vi "Façade 1.vi"(0 "Data In":T4 caption="Données en entrée", 2 "Display State In":T2 caption="État d'affichage en entrée", 3 "Container State":T3 caption="État du conteneur") -> (6 "Data Out":T4 caption="Données en sortie", 7 "Display State Out":T2 caption="État d'affichage en sortie", 8 "Action":T1)   [LabVIEW 2012, in "CommandeX 1.xctl"]
uses:
  CommandeX 1.xctl
  <vilib>/_xctls/Container State.ctl
  <vilib>/_xctls/Action.ctl
  <vilib>/_xctls/XControlSupport.lvlib
panel:
  # "1. Déposez ici les commandes qui constituent l'apparence de la commandeX.\n\n2. Redimensionnez la fenêtre pour l'ajuster aux commandes.\n\n3. Si la taille de la commandeX est fixe, utilisez la page Propriétés du VI ->Apparence de la fenêtre pour empêcher la fenêtre de se redimensionner.\n\n4. Si vous voulez que les commandes se redimensionnent automatiquement quand la commandeX se redimensionne, sélectionnez l'option \"Mettre à l'échelle tous les objets de la face-avant lors du redimensionnement de la fenêtre\" sur la page Fichier ->Propriétés du VI ->Taille de la fenêtre.\n\n5. Affichez le diagramme et traitez les événements des commandes de cette face-avant."
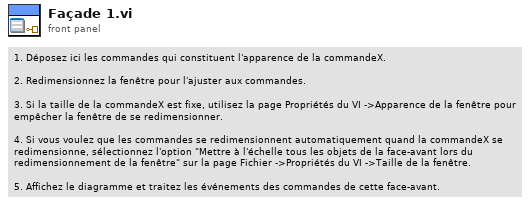
[diagram p1: front panel]
types:
  T1 = typedef "XControlSupport.lvlib/Action.ctl" = cluster{"Data Changed?":bool, "State Changed?":bool, "Action Name":string}
  T2 = typedef "CommandeX 1.xctl/État 1.ctl" = cluster{"Numeric":dbl}
  T3 = typedef "XControlSupport.lvlib/Container State.ctl" = cluster{"Indicator?":bool, "Run Mode?":bool, " Refnum":refnum<vi>}
  T4 = typedef "CommandeX 1.xctl/Données 1.ctl" = dbl
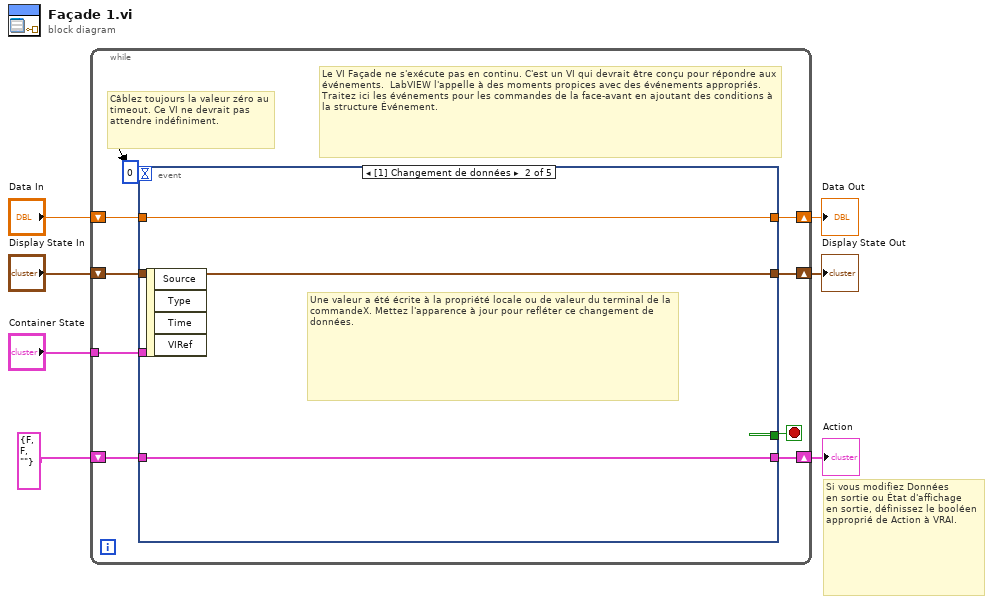
[diagram p0: block diagram]
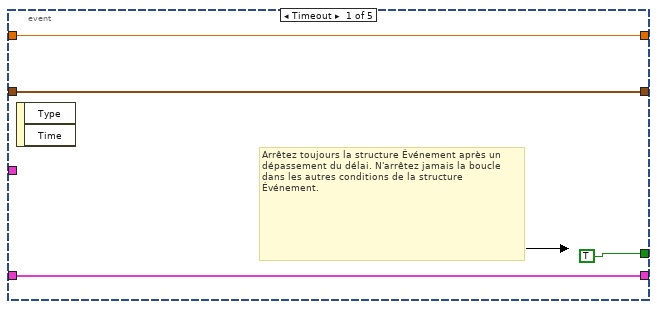
[diagram p2: hidden frame]
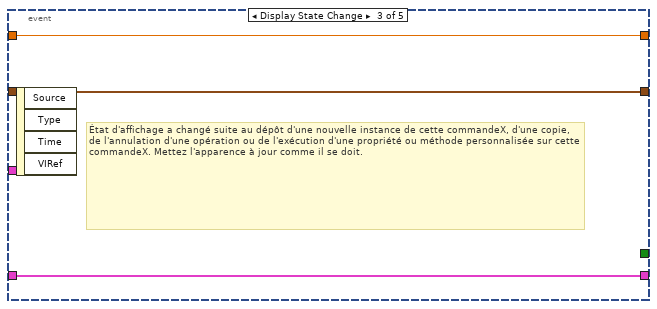
[diagram p3: hidden frame]
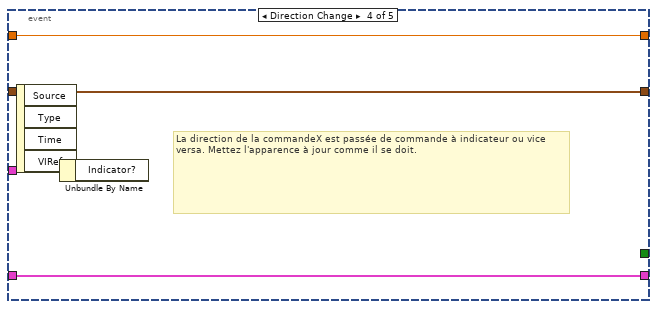
[diagram p4: hidden frame]
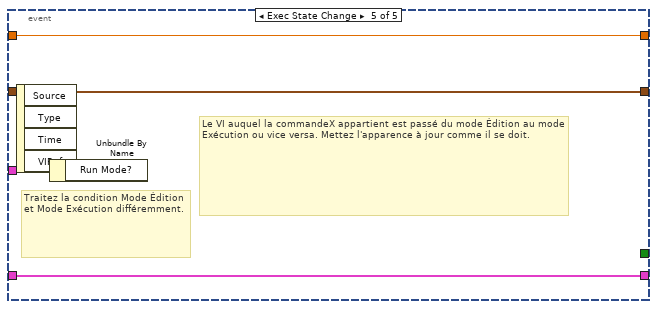
[diagram p5: hidden frame]
diagram:
  # "Si vous modifiez Données\nen sortie ou État d'affichage\nen sortie, définissez le booléen\napproprié de Action à VRAI."
  n1 = while {
    shift-right: [w15] -> w4
    shift-left: "Display State In" -> [w16]
    tunnel: "Container State" -> [w12]
    shift-right: [w10] -> w7
    shift-left: "Data In" -> [w11]
    shift-right: [w8] -> w2
    shift-left: T1 {"Data Changed?"=FALSE, "State Changed?"=FALSE, "Action Name"=""} ("Action") -> [w9]
    stop <- w14 stop-if-true
    # "Le VI Façade ne s'exécute pas en continu. C'est un VI qui devrait être conçu pour répondre aux événements.  LabVIEW l'appelle à des moments propices avec des événements appropriés. Traitez ici les événements pour les commandes de la face-avant en ajoutant des conditions à la structure Événement."
    # "Câblez toujours la valeur zéro au timeout. Ce VI ne devrait pas attendre indéfiniment."
    n2 = event shown="[1] Changement de données" {
      selector: _ -> [_ _ _ _ _]
      dyn-events: _ -> [_ _ _ _ _]
      timeout: 0 -> [_ _ _ _ _]
      tunnel: w16 -> [w18 w22 w26 w29 w33]
      tunnel: [w18 w22 w26 w29 w33] -> w15
      tunnel: [TRUE _ _ _ _] -> w14
      tunnel: w12 -> [_ _ _ w30 w34]
      tunnel: w11 -> [w17 w23 w25 w28 w32]
      tunnel: [w17 w23 w25 w28 w32] -> w10
      tunnel: [w19 w21 w24 w27 w31] -> w8
      tunnel: w9 -> [w19 w21 w24 w27 w31]
      event Timeout {
        # "Arrêtez toujours la structure Événement après un dépassement du délai. N'arrêtez jamais la boucle dans les autres conditions de la structure Événement."
        n3 = event-data() -> ()  [unwired: 1 in, 2 out]
      }
      event Data Change {
        # "Une valeur a été écrite à la propriété locale ou de valeur du terminal de la commandeX. Mettez l'apparence à jour pour refléter ce changement de données."
        n4 = event-data() -> ()  [unwired: 1 in, 4 out]
      }
      event Display State Change {
        # "État d'affichage a changé suite au dépôt d'une nouvelle instance de cette commandeX, d'une copie, de l'annulation d'une opération ou de l'exécution d'une propriété ou méthode personnalisée sur cette commandeX. Mettez l'apparence à jour comme il se doit."
        n5 = event-data() -> ()  [unwired: 1 in, 4 out]
      }
      event Direction Change {
        # "La direction de la commandeX est passée de commande à indicateur ou vice versa. Mettez l'apparence à jour comme il se doit."
        n6 = event-data() -> ()  [unwired: 1 in, 4 out]
        n7 = Unbundle By Name(w30) -> ()  [unwired: 1 out]
      }
      event Exec State Change {
        # "Le VI auquel la commandeX appartient est passé du mode Édition au mode Exécution ou vice versa. Mettez l'apparence à jour comme il se doit."
        # "Traitez la condition Mode Édition et Mode Exécution différemment."
        n8 = event-data() -> ()  [unwired: 1 in, 4 out]
        n9 = Unbundle By Name(w34) -> ()  [unwired: 1 out]
      }
    }
  }
  "Display State Out" <- w4
  "Data Out" <- w7
  "Action" <- w2
